vi "AlliGator Export ROI(s) NLSF Parameters as ASCII File.vi"(7 "AlliGator Ctrl Refnums":T2, 8 "error in (no error)":errorcluster, 10 "All ROIs":bool, 11 "AlliGator IV DVR in":refnum<data-value>) -> (0 "error out":errorcluster, 1 "Message":string, 3 "AlliGator IV DVR out":refnum<data-value>)   [LabVIEW 2021, in "AlliGator Decay Fit Parameter Map.lvlib"]
doc: "Exports Decay Fit Parameter Map data to an ASCII file."
uses:
  AlliGator Decay Fit Parameter Map.lvlib
  Strings/Strings.lvlib
  <userlib>/_OpenG.lib/array/array.llb/openg_array.lvlib
  AlliGator Variables List.ctl
  AlliGator Globals, Variables & Constants.lvlib
  Image/Named ROI Description.ctl
  Image/Image.lvlib
  <vilib>/Utility/file.llb/Write Delimited Spreadsheet (DBL).vi
  Fits/IRF(X)PSED/Decay Fit Parameters & Derived Quantities List.ctl
  Fits/Fits.lvlib
  <userlib>/_OpenG.lib/array/array.llb/Filter 1D Array with Scalar (String)__ogtk.vi
  <vilib>/vision/Image Controls.llb/IMAQ Image.ctl
  Phasor/Phasor Reference Series.ctl
  Phasor/Phasor.lvlib
  Phasor/Calibration Phasor (m, phi).ctl
  Phasor/Phasor (g, s).ctl
  AlliGator Baseline Subtraction Method.ctl
  AlliGator Decay Preprocessing.lvlib
  AlliGator Decay Background Subtraction Info.ctl
  AlliGator Decay Extrapolation Parameters.ctl
  AlliGator Decay Metadata v3.ctl
  AlliGator Phasor Graph.lvlib
  AlliGator Raw Phasor Plot Data v4.ctl
  AlliGator Data Series Type.ctl
  AlliGator Files.lvlib
  AlliGator Internal Variables v2.ctl
  AlliGator Internal Variables.lvlib
  AlliGator FLI Dataset Type.ctl
  Phasor/Phasor Harmonic Data.ctl
  AlliGator Phasor Multi-Harmonic Data.ctl
  AlliGator Phasor Plot.lvlib
  AlliGator Displayed Image.ctl
  AlliGator Source Image.lvlib
  Fits/IRF(X)PSED/Decay Fit Parameters In List.ctl
  AlliGator Decay Fit Parameter Constraints 2.ctl
  AlliGator Decay Fit.lvlib
  Fits/Decay Convolution/Decay Model.ctl
  Fits/Residual Type.ctl
  Fits/Fit Calculation Method.ctl
  Fits/Non-linear Fitting Algorithm.ctl
  AlliGator Decay Fit Options & Parameters v2.ctl
  Fits/IRF(X)PSED/Fit Weights Type.ctl
  AlliGator Gate Image Set.ctl
  AlliGator Gate Arithmetic.ctl
  AlliGator Settings.lvlib
  AlliGator Dataset Channel.ctl
  AlliGator Dual-Channel Datasets.lvlib
  AlliGator Registered Events Ctrl Refnums.ctl
  AlliGator GUI.lvlib
  AlliGator Dataset Ctrl Refnums.ctl
  Phasor/Phasor Calibration Type.ctl
  AlliGator Phasor Graph Ctrl Refnums.ctl
  AlliGator Phasor Plot Ctrl Refnums.ctl
  AlliGator State Indicator.ctl
  AlliGator Other Ctrl Refnums.ctl
  Histograms/Histogram Bin Position.ctl
  Histograms/Histogram Window.lvlib
  Histograms/Histogram Bin Option.ctl
  Histograms/Linear Histogram Options.ctl
  AlliGator Image Histogram Control Refnums.ctl
  AlliGator Decay Fit Map Control Refnums.ctl
  AlliGator Ctrl Refnums.ctl
  Graphs/XY Graph/XY Graph Plot Shift Method.ctl
  Graphs/XY Graph/XY Graph Add-Ons.lvlib
  Graphs/XY Graph/XY Graph Plot Shift Parameters.ctl
  AlliGator Decay Preprocessing Parameters.ctl
  Phasor/Phasor Standard Deviation Options.ctl
  Phasor/Phasor Calibration Map v2.ctl
  Fits/Non-linear Fitting Method v2.ctl
  Fits/IRF(X)PSED/Decay Fit Options v2.ctl
  Fits/IRF(X)PSED/MLE Baseline Offset Type.ctl
  AlliGator Parameter Maps Data.ctl
  AlliGator Main Window Tabs.ctl
panel:
  in  "Fit Parameter (for diagram use)":T1
  # "see the AlliGator License on the block diagram (Ctrl+E or Window:Show Block Diagram)"
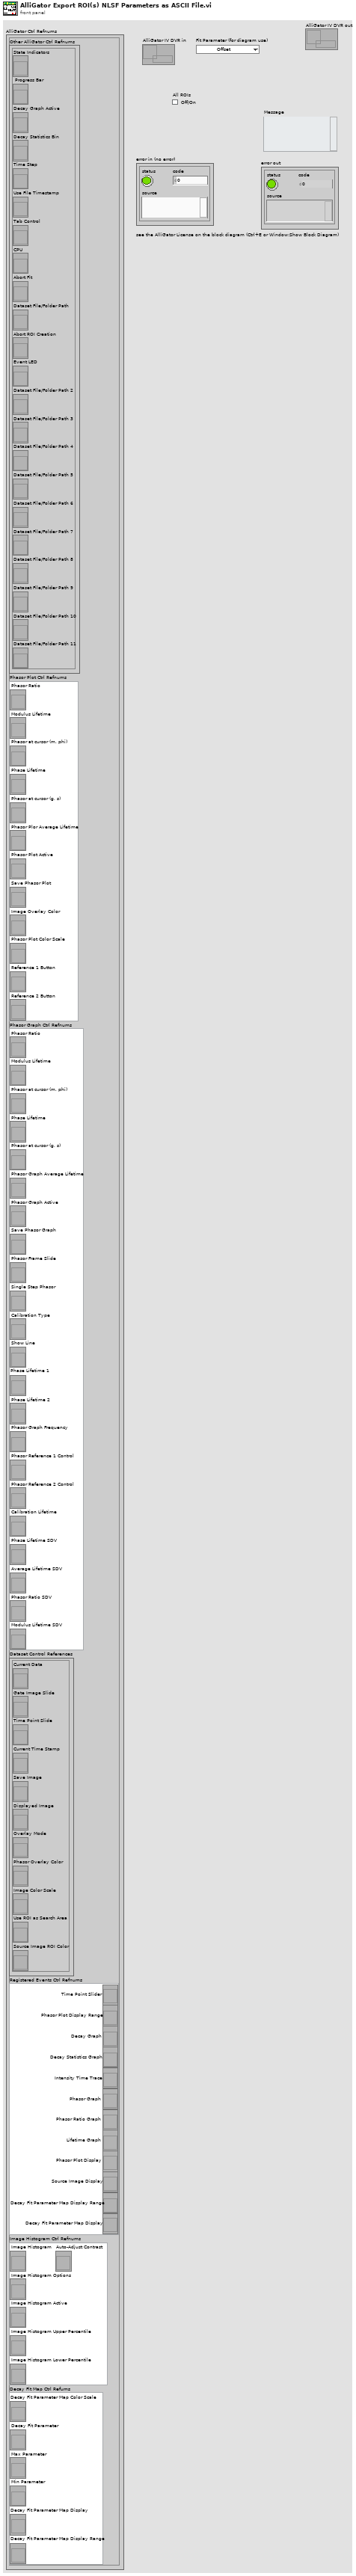
[diagram p1: front panel]
types:
  T1 = typedef "Fits.lvlib/Decay Fit Parameters & Derived Quantities List.ctl" = enum16{"Offset", "Baseline", "A_1", "tau_1", "A_2", "tau_2", "<tau>_a", "f1_a", "f2_a", "<tau>_i", "f1_i", "f2_i", "-", "R^2", "Chi^2"}
  T2 = typedef "AlliGator GUI.lvlib/AlliGator Ctrl Refnums.ctl" = cluster{"Other AlliGator Ctrl Refnums":T3, "Phasor Plot Ctrl Refnums":T4, "Phasor Graph Ctrl Refnums":T5, "Dataset Control References":T6, "Registered Events Ctrl Refnums":T7, "Image Histogram Ctrl Refnums":T8, "Decay Fit Map Ctrl Refums":T9}
  T3 = typedef "AlliGator GUI.lvlib/AlliGator Other Ctrl Refnums.ctl" = cluster{"State Indicators":refnum<vi>, " Progress Bar":refnum<vi>, "Decay Graph Active":refnum<vi>, "Decay Statistics Bin":refnum<vi>, "Time Step":refnum<vi>, "Use File Timestamp":refnum<vi>, "Tab Control":refnum<vi>, "CPU":refnum<vi>, "Abort Fit":refnum<vi>, "Dataset File/Folder Path":refnum<vi>, "Abort ROI Creation":refnum<vi>, "Event LED":refnum<vi>, "Dataset File/Folder Path 2":refnum<vi>, "Dataset File/Folder Path 3":refnum<vi>, "Dataset File/Folder Path 4":refnum<vi>, "Dataset File/Folder Path 5":refnum<vi>, "Dataset File/Folder Path 6":refnum<vi>, "Dataset File/Folder Path 7":refnum<vi>, "Dataset File/Folder Path 8":refnum<vi>, "Dataset File/Folder Path 9":refnum<vi>, "Dataset File/Folder Path 10":refnum<vi>, "Dataset File/Folder Path 11":refnum<vi>}
  T4 = typedef "AlliGator GUI.lvlib/AlliGator Phasor Plot Ctrl Refnums.ctl" = cluster{"Phasor Ratio":refnum<vi>, "Modulus Lifetime":refnum<vi>, "Phasor at cursor (m, phi)":refnum<vi>, "Phase Lifetime":refnum<vi>, "Phasor at cursor (g, s)":refnum<vi>, "Phasor Plor Average Lifetime":refnum<vi>, "Phasor Plot Active":refnum<vi>, "Save Phasor Plot":refnum<vi>, "Image Overlay Color":refnum<vi>, "Phasor Plot Color Scale":refnum<vi>, "Reference 1 Button":refnum<vi>, "Reference 2 Button":refnum<vi>}
  T5 = typedef "AlliGator GUI.lvlib/AlliGator Phasor Graph Ctrl Refnums.ctl" = cluster{"Phasor Ratio":refnum<vi>, "Modulus Lifetime":refnum<vi>, "Phasor at cursor (m, phi)":refnum<vi>, "Phase Lifetime":refnum<vi>, "Phasor at cursor (g, s)":refnum<vi>, "Phasor Graph Average Lifetime":refnum<vi>, "Phasor Graph Active":refnum<vi>, "Save Phasor Graph":refnum<vi>, "Phasor Frame Slide":refnum<vi>, "Single Step Phasor":refnum<vi>, "Calibration Type":refnum<vi>, "Show Line":refnum<vi>, "Phase Lifetime 1":refnum<vi>, "Phase Lifetime 2":refnum<vi>, "Phasor Graph Frequency":refnum<vi>, "Phasor Reference 1 Control":refnum<vi>, "Phasor Reference 2 Control":refnum<vi>, "Calibration Lifetime":refnum<vi>, "Phase Lifetime SDV":refnum<vi>, "Average Lifetime SDV":refnum<vi>, "Phasor Ratio SDV":refnum<vi>, "Modulus Lifetime SDV":refnum<vi>}
  T6 = typedef "AlliGator GUI.lvlib/AlliGator Dataset Ctrl Refnums.ctl" = cluster{"Current Data":refnum<vi>, "Gate Image Slide":refnum<vi>, "Time Point Slide":refnum<vi>, "Current Time Stamp":refnum<vi>, "Save Image":refnum<vi>, "Displayed Image":refnum<vi>, "Overlay Mode":refnum<vi>, "Phasor Overlay Color":refnum<vi>, "Image Color Scale":refnum<vi>, "Use ROI as Search Area":refnum<vi>, "Source Image ROI Color":refnum<vi>}
  T7 = typedef "AlliGator GUI.lvlib/AlliGator Registered Events Ctrl Refnums.ctl" = cluster{"Time Point Slider":refnum<vi>, "Phasor Plot Display Range":refnum<vi>, "Decay Graph":refnum<vi>, "Decay Statistics Graph":refnum<vi>, "Intensity Time Trace":refnum<vi>, "Phasor Graph":refnum<vi>, "Phasor Ratio Graph":refnum<vi>, "Lifetime Graph":refnum<vi>, "Phasor Plot Display":refnum<vi>, "Source Image Display":refnum<vi>, "Decay Fit Parameter Map Display Range":refnum<vi>, "Decay Fit Parameter Map Display":refnum<vi>}
  T8 = typedef "AlliGator GUI.lvlib/AlliGator Image Histogram Control Refnums.ctl" = cluster{"Image Histogram":refnum<vi>, "Image Histogram Options":refnum<vi>, "Image Histogram Active":refnum<vi>, "Image Histogram Upper Percentile":refnum<vi>, "Image Histogram Lower Percentile":refnum<vi>, "Auto-Adjust Contrast":refnum<vi>}
  T9 = typedef "AlliGator Decay Fit Parameter Map.lvlib/AlliGator Decay Fit Map Control Refnums.ctl" = cluster{"Decay Fit Parameter Map Color Scale":refnum<vi>, "Decay Fit Parameter":refnum<vi>, "Max Parameter":refnum<vi>, "Min Parameter":refnum<vi>, "Decay Fit Parameter Map Display":refnum<vi>, "Decay Fit Parameter Map Display Range":refnum<vi>}
  T10 = typedef "Image.lvlib/Named ROI Description.ctl" = cluster{"ROI Descriptor":T11, "ROI Name":string, "Overlay Color":u32}
  T11 = typedef "ROI Descriptor" = cluster{"Global Rectangle":i32[], "Contours":cluster{"ID":enum32{"External", "Internal"}, "Type":u32, "Coordinates":i32[]}[]}
  T12 = typedef "AlliGator Globals, Variables & Constants.lvlib/AlliGator Variables List.ctl" = enum16{"---- GUI ----", "GUI:Initialization Status", "GUI:State Indicators Refnum", "GUI:Original AlliGator Menu Items", "GUI:Current Action Loop State", "GUI:Script in progress", "GUI:Playback", "GUI:Loop Playback", "GUI:Search ROI Used", "GUI:Search ROI", "Decay Graph Max Legend Size", "Intensity Graph Max Legend Size", "Decay Statistics Graph Max Legend Size", "Phasor Graph Max Legend Size", "Phasor Ratio Graph Max Legend Size", "Lifetime Graph Max Legend Size", "---- Files ----", "Files:Export Dataset Frames as Individual Files", "Files:Show Batch Export Help Balloons", "Files:Frames in Dataset", "Files:ptu File Frame Start Indices", "Files:Current Frame in Dataset", "Files:Current Frame Timestamp", "Files:Dataset Loaded", "Files:Dataset Metadata", "Files:Dataset Channel", "Files:Dataset Data Description", "Files:Background Dataset Metadata", "Files:Background Dataset Channel", "Files:Background Dataset Data Description", "Files:Background File Subtraction", "Files:Background File Path", "Files:Background File Pile-up Correction", "Files:Background File Pixel Well Capacity", "Files:Background File Scaling Factor", "Files:Current Dataset Load Settings", "Files:Dataset Path", "Files:ICCD-specific Information", "Files:Macrotime Gate Separation", "------ Python Plugins ------", "Python Plugins:Information", "Python Plugins:Python Session", "Python Plugins:Valid Python Session?", "---- Source Image ----", "Source Image:ROIs", "Source Image:Current ROI", "Source Image:ROI Event Refnum", "X_Source Image Display Range", "X_Source Image Palette Information", "X_Type of Displayed Image", "X_Time Gate Slider", "Source Image:Palette List", "Source Image:Scale", "Source Image:ROI Overlay Color", "Source Image:Overlay to Erase", "Source Image:Is Displayed Image Accumulated", "Source Image:White Light Image Modified", "Source Image:Mask Image Modified", "---- Image Profile Window ----", "Image Profile:Overlay ROI in Source Image", "Image Profile:Window Event Refnum", "Image Profile:IntensityType", "Image Profile:Intensity Average Type", "Image Profile:Intensity-weighted SDV", "Image Profile:Box Profile Type", "Image Profile:Window Open", "Image Profile:Plotted Fit Parameter", "------ Phasor Graph -------", "Phasor Graph:Show Line", "---- Phasor Plot ---", "Phasor Plot:Parameters Changed", "Phasor Plot:FLI Dataset Modified since last Calculation", "Phasor Harmonics Data", "Selected Phasor Harmonics", "Phasor Harmonic Manager Event Refnum", "Phasor Plot:ROIs", "Phasor Plot:Current ROI", "Phasor Plot:ROI Event Refnum", "Phasor Plot:Image Reference Points", "Phasor Plot:Computed", "Phasor Plot:Palette Information", "Phasor Plot:Palette List", "Phasor Plot:Phasor Ratio Palette Information", "Phasor Plot:Phasor Ratio Palette List", "Phasor Plot:Image Scale", "Phasor Plot:Image Overlay to Erase", "Phasor Plot:Image Elements to Update", "Phasor Plot:Current Calculation Parameters", "Phasor Plot:Current Calibration Options", "Phasor Plot:Reset Cumulated Phasor Plot", "Phasor Plot:Reference 1", "Phasor Plot:Lifetime Reference 1", "Phasor Plot:Reference 1 Frequency", "Phasor Plot:Reference 2", "Phasor Plot:Lifetime Reference 2", "Phasor Plot:Reference 2 Frequency", "---- Decay Analysis ----", "Number of Selected Decays to Fit", "LS Fit Results", "LAR Fit Results", "BS Fit Results", "Last Decay Max - Min", "Best Fit Parameters", "Best Fit Parameter Names", "Actual Size X", "Actual Size Y", "Binning X", "Binning Y", "Actual # Gates", "Dataset Number", "Gates to...", "Gates Skipped", "Gates to keep", "Gate Step", "Gate Separation", "Reversed Gates", "Pile-up Correction", "Pixel Well Capacity", "Background Subtracted", "Background Subtraction Method", "Background Definition Range", "Background File (deprecated)", "Number of Dataset Accumulated", "Array of Accumulated Dataset Paths", "Do Averaged Datasets", "Destination File Path", "Process Plot Target", "Use 1/D as Phasor Frequency", "---- Decay Fit Parameter Map -----", "Decay Fit Parameter Map:Palette Information", "Decay Fit Parameter Map:Palette List", "------- Local Decay Window ---------", "Local Decay Graph Window:Event Refnum", "Local Decay Graph Window:Use normalized IRF for convolution", "----- Miscellaneous ----", "Misc:Skippable Dialog Windows Status"}
  T13 = typedef "AlliGator Internal Variables.lvlib/AlliGator Internal Variables v2.ctl" = cluster{"Displayed Image":T14, "White Light Image":T14, "Mask Image":T14, "ROI Mask Image":T14, "Current Dataset Images 1":T15, "Background Dataset Images 1":T15, "Current Dataset Images 2":T15, "Background Dataset Images 2":T15, "Current Dataset Arithmetic Images":T15, "Accumulated Dataset Images 1":T15, "Accumulated Dataset Images 2":T15, "Accumulated Dataset Arithmetic Images":T15, "Phasor Plot Image":T14, "Decay Fit Parameter Map Image":T14, "Single Data Point Path":path, "White Light Image Path":path, "Mask Image Path":path, "Time-Series Folder":path, "[Time-Series Paths]":path[], "Current Dataset":i32, "Single Dataset Type":T16, "Current Folder":string, "AlliGator Data Series Type":T17, "# Datasets":i32, "Dual-Channel Dataset":bool, "Selected Channel Name":string, "Dataset Channel":T18, "Channel Arithmetic":T19, "Dual-Channel Background Dataset":bool, "Background Channel":T18, "Dual-Channel Accumulated Dataset":bool, "Start Time":dbl, "[Time-Series Timestamps]":dbl[], "[Intensity Corrections]":dbl[], "Time Series Script":bool, "Type of Displayed Image":T20, "Gate Image Slide":u16, "# Gates":i32, "ROIs":T10[], "ROI Decay":cluster{"t Array":dbl[], "I Array":dbl[]}, "Valid Decay":bool, "Decay  Metadata":T21, "Reference Decay Plot Name":string, "Reference Decay":cluster{"t Array":dbl[], "I Array":dbl[]}, "Decay Shift Plot":cluster{"Time Stamps":dbl[], "Decay Shifts":dbl[]}, "[Decays Max Values]":sgl[], "[Decays Min Values]":sgl[], "Calibration Phasor":T27, "Calibration Phasor Series":T28, "Phasor Calibration Map":T29, "Calibration Map MD5 Digest":string, "Last Raw Phasor":T30, "Last Calibrated Phasor":T30, "Last Calibrated Phasor SDV":T30, "Phasor Graph:Phasor Plot":cluster{"g Array":dbl[], "s Array":dbl[]}, "Phasor Graph:Phasor SDV Plot":cluster{"g Array":dbl[], "s Array":dbl[]}, "[Phasor Graph:Raw Phasor Plots]":T31[], "Phasor Plot locked to Ref 1":i32, "[Phasor Plot(s) locked to Ref 1]":i32[], "[Phasor Plot(s) locked to Ref 2]":i32[], "[Pixel Phasors]":T30[], "[[Sum Image]]":dbl[][], "[[CSG Phasors]]":csg[][], "[[Valid Pixel?]]":bool[][], "I/m/phi Dataset":cluster{"I/m/phi Dataset?":bool, "Base Frequency":dbl[unit], "Harmonic Orders":u8[]}, "Multi Phasor Plot Data":T33, "Decay Fit Options & Parameters":T35, "Fit Options: Decay Preprocessing Parameters":T46, "Fit Options: Reference Decay":cluster{"t Array":dbl[], "I Array":dbl[]}, "Is Full Image Parameters Map":bool, "Is Single-Pixels Parameters Map":bool, "NLSF Parameters Map X Resolution":i32, "NLSF Parameters Map Y Resolution":i32, "[Single Decay Fit Parameters]":dbl[], "Fit Model":T37, "[[Multiple Decays Fit Parameters]]":dbl[][], "[[Multiple Decays Fit Parameter SDVs]]":dbl[][], "[[IRFs]]":dbl[][], "IRF Array Time Axis":dbl[], "Decay Array Time Axis":dbl[], "[Decay Fit Parameter Names]":T1[], "[[Phasor Ratios]]":dbl[][], "[[Average Lifetimes]]":dbl[][], "Amplitude Weighted Average Lifetime":bool, "[Decay Sum]":dbl[], "Parameter Maps":T47[], "[[User-defined Quantities]]":dbl[][], "User-defined Quantity":string}
  T14 = typedef "IMAQ Image.ctl" = refnum<image>
  T15 = typedef "AlliGator Internal Variables.lvlib/AlliGator Gate Image Set.ctl" = cluster{"SGL Image Max":T14, "SGL Image Sum":T14, "SGL Gate Images":T14[], "SGL Image Min":T14}
  T16 = typedef "AlliGator Files.lvlib/AlliGator FLI Dataset Type.ctl" = enum16{"HDF5 FLI Dataset", "Gate Image Folder", ".sdt FLI Dataset (Becker & Hickl)", ".ptu FLI Dataset (PicoQuant)", "SS1 FLI Dataset", "SS2 FLI Dataset", "I/m/phi Dataset", ".bin FLI Dataset (PicoQuant Binned)", ".bin FLI Dataset (Piccolo Binned)"}
  T17 = typedef "AlliGator Files.lvlib/AlliGator Data Series Type.ctl" = enum16{"Not a Supported Series", "Gate Images Folder Series", "SwissSPAD 2 Dataset Series", "B&H FLI Dataset Series", "PicoQuant PTU FLI Dataset Series", "PicoQuant BIN FLI Dataset Series", "Piccolo hist BIN FLI Dataset Series", "HDF5 FLI Dataset Series"}
  T18 = typedef "AlliGator Dual-Channel Datasets.lvlib/AlliGator Dataset Channel.ctl" = enum16{"G2", "INT"}
  T19 = typedef "AlliGator Settings.lvlib/AlliGator Gate Arithmetic.ctl" = enum16{"None", "INT-G2", "G2/INT*<INT>", "(1 - G2/INT)*<INT>"}
  T20 = typedef "AlliGator Source Image.lvlib/AlliGator Displayed Image.ctl" = enum16{"Single Gate", "Sum of All Gates", "Max of All Gates", "Min of All Gates", "-", "White Ligth Image", "Mask Image"}
  T21 = typedef "AlliGator Phasor Graph.lvlib/AlliGator Decay Metadata v3.ctl" = cluster{"ROI Descriptor":T11, "ROI Center":cluster{"X":i32, "Y":i32}, "Decay Background Subtraction Info":T22, "Decay Reverted":bool, "Decay Smoothened":bool, "Decay Straightened":bool, "Fitted Tau (Decay Straightening)":dbl, "Decay Shift Parameters":T24, "Decay Shifted":bool, "Decay Extrapolated":bool, "Decay Extrapolation Parameters":T26, "Decay Normalized":bool, "Fold Decay":bool, "# Folds":u32}
  T22 = typedef "AlliGator Decay Analysis.lvlib/AlliGator Decay Preprocessing.lvlib/AlliGator Decay Background Subtraction Info.ctl" = cluster{"Laser Period":dbl[unit], "Gate Duration":dbl[unit], "Baseline Subtraction Method":T23, "Background Definition Range":cluster{"Min Gate":dbl[unit], "Max Gate":dbl[unit]}, "Total Intensity w/o Bkgd Subtraction":dbl, "Bkgd-subtracted Intensity (exp)":dbl, "# Data Points":i32, "Background/Gate":dbl, "Fitted Lifetime":dbl[unit], "Bkgd-subtracted Intensity (theo)":dbl}
  T23 = typedef "AlliGator Decay Analysis.lvlib/AlliGator Decay Preprocessing.lvlib/AlliGator Baseline Subtraction Method.ctl" = enum16{"Mean", "Min", "Square Gated Single-Exponential", "File", "Constant"}
  T24 = typedef "XY Graph Add-Ons.lvlib/XY Graph Plot Shift Parameters.ctl" = cluster{"Type":T25, "Shift":dbl[unit], "Threshold":dbl, "Rotate":bool}
  T25 = typedef "XY Graph Add-Ons.lvlib/XY Graph Plot Shift Method.ctl" = enum16{"Default", "CFD", "Threshold", "Cross-Correlation"}
  T26 = typedef "AlliGator Decay Analysis.lvlib/AlliGator Decay Preprocessing.lvlib/AlliGator Decay Extrapolation Parameters.ctl" = cluster{"Additional Points":u32, "Head Fraction":dbl, "Fitted Tau":dbl, "Use Periodicity":bool, "Use Cursors":bool, "Tail Fraction":dbl}
  T27 = typedef "Phasor.lvlib/Calibration Phasor (m, phi).ctl" = cluster{"m":dbl, "phi":dbl, "Phasor Frequency":dbl[unit], "Reference Lifetime":dbl[unit]}
  T28 = typedef "Phasor.lvlib/Phasor Reference Series.ctl" = cluster{"m Array":dbl[], "phi Array":dbl[], "Phasor Frequency":dbl[unit], "Calibration Lifetime":dbl[unit]}
  T29 = typedef "Phasor.lvlib/Phasor Calibration Map v2.ctl" = cluster{"Phasor Frequency":dbl[unit], "Calibration Lifetime":dbl[unit], "ROI Centers":cluster{"X":i32, "Y":i32}[], "ROI Descriptors":T11[], "Map Resolution X":i32, "Map Resolution Y":i32, "z Array":cdb[]}
  T30 = typedef "Phasor.lvlib/Phasor (g, s).ctl" = cluster{"g":dbl, "s":dbl}
  T31 = typedef "AlliGator Phasor Graph.lvlib/AlliGator Raw Phasor Plot Data v4.ctl" = cluster{"Phasor Plot Name":string, "Raw Phasor Plot":T30[], "Phasor Frequency":dbl[unit], "[Decay Metadata]":T21[], "Raw Phasor Plot SDV":T30[], "Phasor SDV Options":T32, "[Calibration Phasor]":T27[]}
  T32 = typedef "Phasor.lvlib/Phasor Standard Deviation Options.ctl" = cluster{"Compute Estimated SDV":bool, "# Replicas":u32, "Use Estimated Average Phasor":bool}
  T33 = typedef "AlliGator Phasor Plot.lvlib/AlliGator Phasor Multi-Harmonic Data.ctl" = cluster{"Base Frequency":dbl[unit], "# Harmonics":u8, "Harmonic Orders":u8[], "Phasor Plot Settings Checksum":u64, "Phasor Harmonic Data Array":T34[]}
  T34 = typedef "Phasor.lvlib/Phasor Harmonic Data.ctl" = cluster{"Phasor Harmonic Name":string, "Phasor Plot Settings Checksum":u64, "Phasor Frequency":dbl[unit], "Base Frequency":dbl[unit], "Harmonic Order":u8, "Phasor Plot Parameters":string, "Phasor Array [[CSG]]":csg[][], "Dataset File Path":path}
  T35 = typedef "AlliGator Decay Fit Parameter Map.lvlib/AlliGator Decay Fit Options & Parameters v2.ctl" = cluster{"SYNC Period":dbl[unit], "Fit Options":T36, "Fit Parameter Constraints":T43[], "MLE Baseline Offset":dbl, "MLE Baseline Offset Type":T45}
  T36 = typedef "Fits.lvlib/Decay Fit Options v2.ctl" = cluster{"Show Fit Residuals":bool, "Fit Model":T37, "Residual Type":T38, "Max Decay Percentile":dbl, "Min Decay Percentile":dbl, "Show Full Decay":bool, "Weights":T39, "Fitting Method":T40, "Compute Parameter Uncertainties":bool, "Periodic Boundaries":bool, "Model Calculation":T41, "Period":dbl[unit], "Termination Criteria":cluster{"Max Iterations":i32, "Max Function Calls":i32, "Max Time":dbl[unit], "Function Tolerance":dbl, "Parameter Tolerance":dbl, "Gradient Tolerance":dbl, "Min Lambda":dbl, "Max Lambda":dbl, "Initial Tick Count":u32}, "Offset Resolution":dbl[unit], "Use Local IRF":bool, "Fitting Algorithm":T42}
  T37 = typedef "Fits.lvlib/Decay Model.ctl" = enum16{"1-Exponential", "2-Exponentials"}
  T38 = typedef "Fits.lvlib/Residual Type.ctl" = enum16{"Standard", "Normalized", "Reduced"}
  T39 = typedef "Fits.lvlib/Fit Weights Type.ctl" = enum16{"Unweighted", "1/Variance", "Best of All"}
  T40 = typedef "Fits.lvlib/Non-linear Fitting Method v2.ctl" = enum16{"Least Square", "Least Absolute Residual", "Bisquare", "MLE", "-", "Best of All"}
  T41 = typedef "Fits.lvlib/Fit Calculation Method.ctl" = enum16{"Simulation", "Convolution", "Integration"}
  T42 = typedef "Fits.lvlib/Non-linear Fitting Algorithm.ctl" = enum16{"Levenberg-Marquardt", "Trust-Region Dogleg"}
  T43 = typedef "AlliGator Decay Analysis.lvlib/AlliGator Decay Fit.lvlib/AlliGator Decay Fit Parameter Constraints 2.ctl" = cluster{"Fit Parameter":T44, "Min Value":dbl, "Max Value":dbl, "Global":bool, "Used":bool}
  T44 = typedef "Fits.lvlib/Decay Fit Parameters In List.ctl" = enum16{"Offset", "Baseline", "A_1", "tau_1", "A_2", "tau_2"}
  T45 = typedef "Fits.lvlib/MLE Baseline Offset Type.ctl" = enum32{"Absolute", "Percentage"}
  T46 = typedef "AlliGator Decay Analysis.lvlib/AlliGator Decay Preprocessing.lvlib/AlliGator Decay Preprocessing Parameters.ctl" = cluster{"Background Subtraction":bool, "Straighten Decay":bool, "Reverse Gates":bool, "1-Normalized Decay":bool, "Smoothen Decay":bool, "Smoothing Parameter":dbl, "Shift Decay":bool, "Decay Shift Parameters":T24, "Extrapolate Decay":bool, "Additional Points":u32, "Head Fraction":dbl, "Pixel-Normalize Decay":bool, "Use Periodicity":bool, "Use Cursors":bool, "Tail Fraction":dbl, "Use Decay Pre-Processing":bool, "Fold Decay":bool, "# Folds":u32, "[0-1]-Normalized Decay":bool}
  T47 = typedef "AlliGator Parameter Maps Data.ctl" = cluster{"Map Set Name":string, "[Parameter Names]":string[], "[[Parameters]]":dbl[][], "[[Parameter SDVs]]":dbl[][], "Decay Array Time Axis":dbl[], "[[IRFs]]":dbl[][], "IRF Array Time Axis":dbl[]}
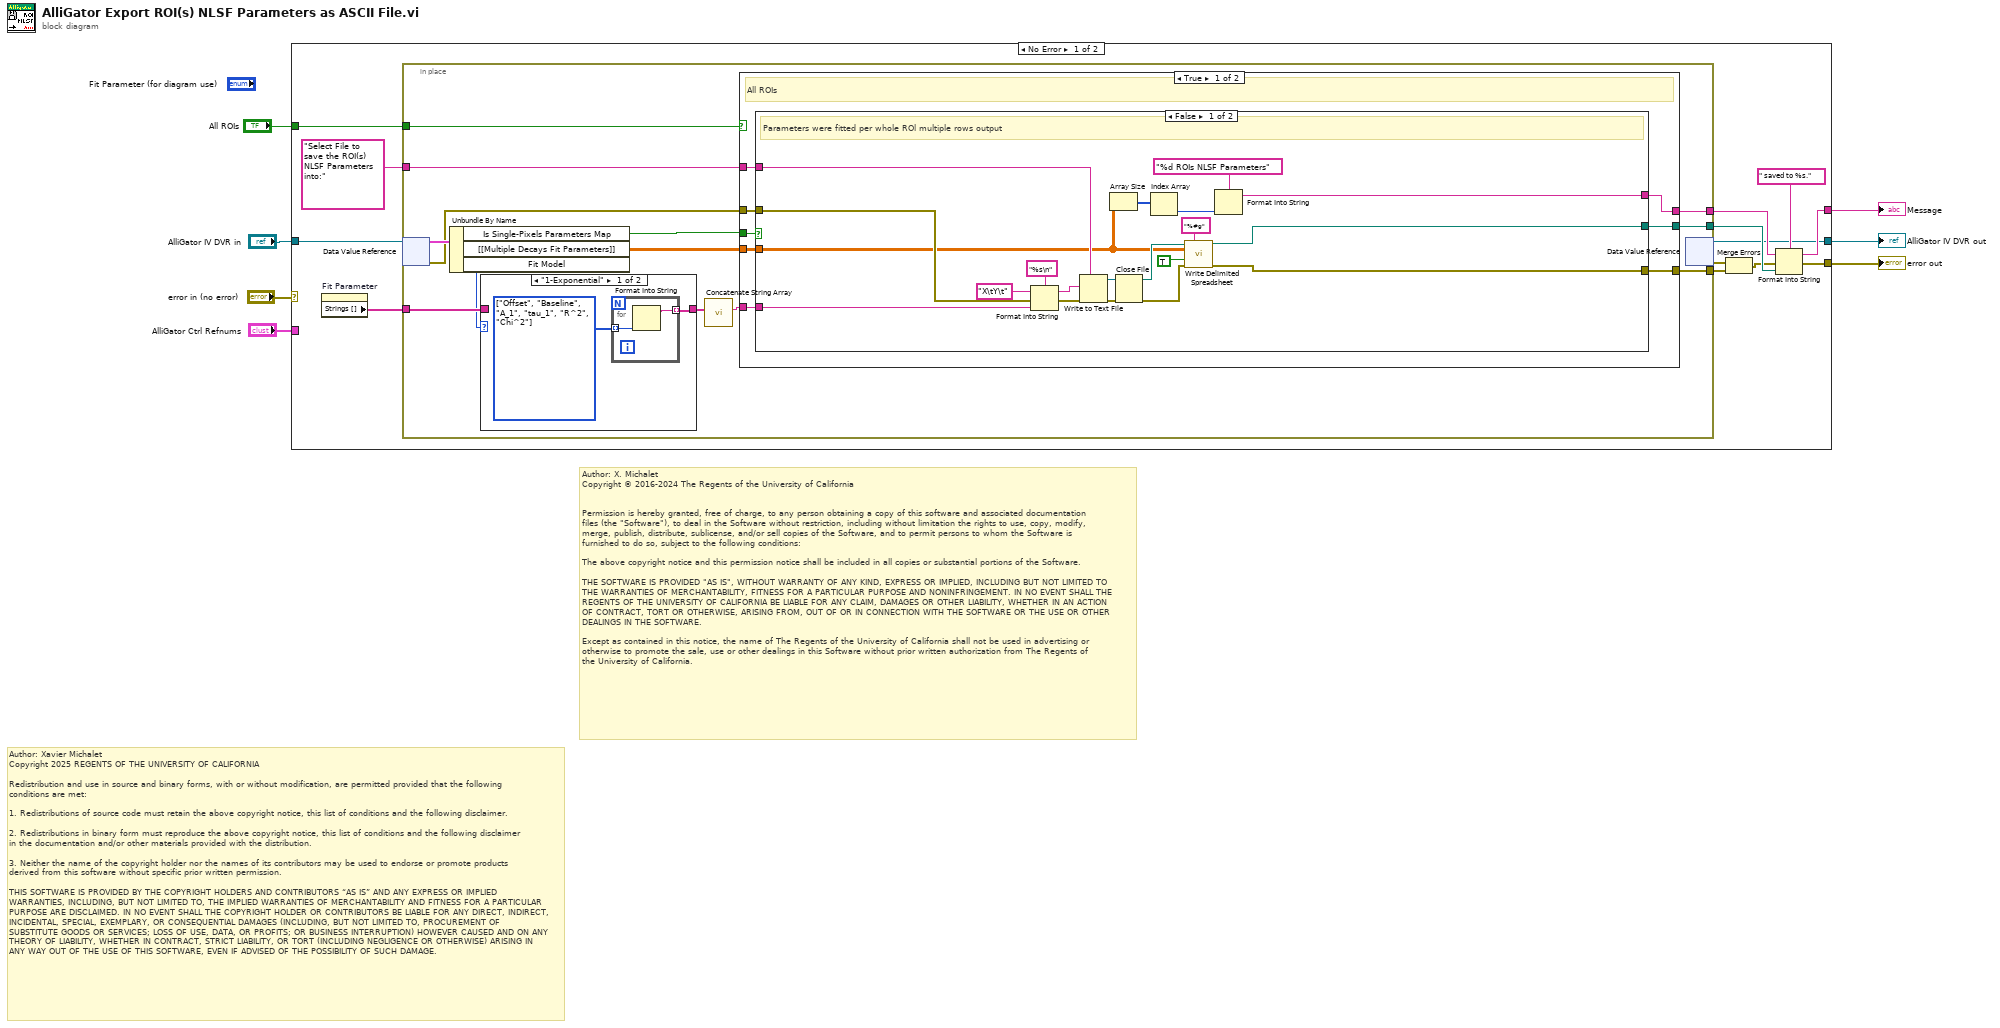
[diagram p0: block diagram]
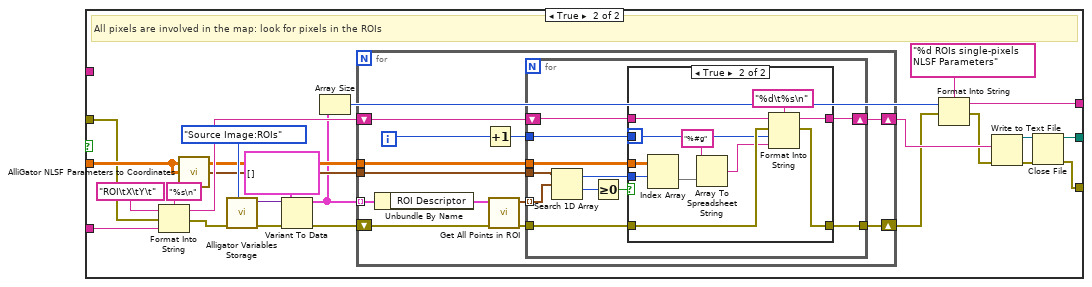
[diagram p2: hidden frame]
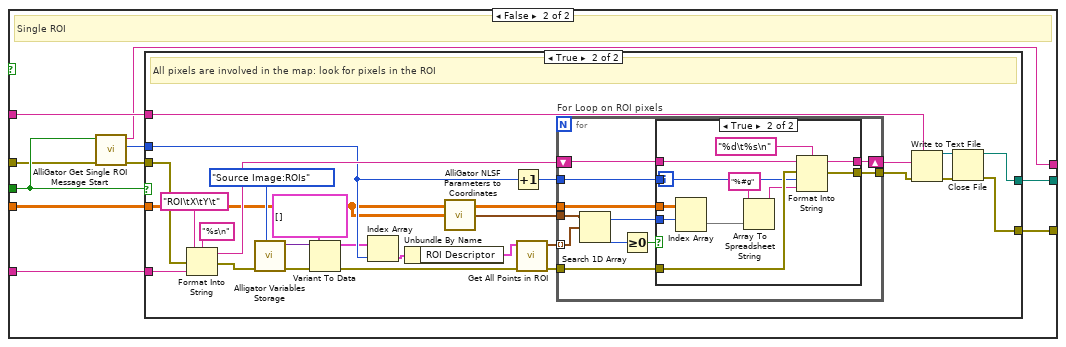
[diagram p4: hidden frame]
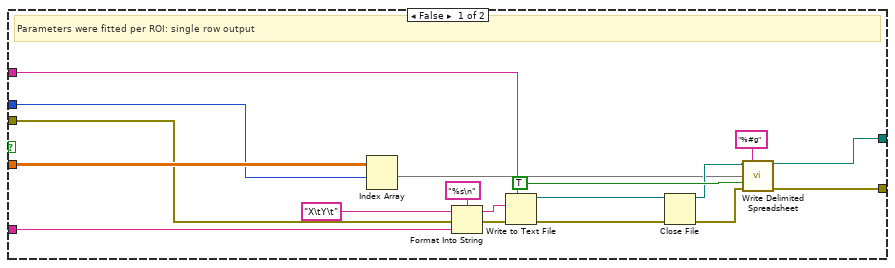
[diagram p5: hidden frame]
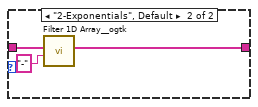
[diagram p7: hidden frame]
diagram:
  # "Author: Xavier Michalet\nCopyright 2025 REGENTS OF THE UNIVERSITY OF CALIFORNIA\n\nRedistribution and use in source and binary forms, with or without modification, are permitted provided that the following conditions are met:\n\n1. Redistributions of source code must retain the above copyright notice, this list of conditions and the following disclaimer.\n\n2. Redistributions in binary form must reproduce the above copyright notice, this list of conditions and the following disclaimer in the documentation and/or other materials provided with the distribution.\n\n3. Neither the name of the copyright holder nor the names of its contributors may be used to endorse or promote products derived from this software without specific prior written permission.\n\nTHIS SOFTWARE IS PROVIDED BY THE COPYRIGHT HOLDERS AND CONTRIBUTORS “AS IS” AND ANY EXPRESS OR IMPLIED WARRANTIES, INCLUDING, BUT NOT LIMITED TO, THE IMPLIED WARRANTIES OF MERCHANTABILITY AND FITNESS FOR A PARTICULAR PURPOSE ARE DISCLAIMED. IN NO EVENT SHALL THE COPYRIGHT HOLDER OR CONTRIBUTORS BE LIABLE FOR ANY DIRECT, INDIRECT, INCIDENTAL, SPECIAL, EXEMPLARY, OR CONSEQUENTIAL DAMAGES (INCLUDING, BUT NOT LIMITED TO, PROCUREMENT OF SUBSTITUTE GOODS OR SERVICES; LOSS OF USE, DATA, OR PROFITS; OR BUSINESS INTERRUPTION) HOWEVER CAUSED AND ON ANY THEORY OF LIABILITY, WHETHER IN CONTRACT, STRICT LIABILITY, OR TORT (INCLUDING NEGLIGENCE OR OTHERWISE) ARISING IN ANY WAY OUT OF THE USE OF THIS SOFTWARE, EVEN IF ADVISED OF THE POSSIBILITY OF SUCH DAMAGE."
  # "Author: X. Michalet\nCopyright © 2016-2024 The Regents of the University of California\n \n\nPermission is hereby granted, free of charge, to any person obtaining a copy of this software and associated documentation files (the \"Software\"), to deal in the Software without restriction, including without limitation the rights to use, copy, modify, merge, publish, distribute, sublicense, and/or sell copies of the Software, and to permit persons to whom the Software is furnished to do so, subject to the following conditions:\n\nThe above copyright notice and this permission notice shall be included in all copies or substantial portions of the Software.\n\nTHE SOFTWARE IS PROVIDED \"AS IS\", WITHOUT WARRANTY OF ANY KIND, EXPRESS OR IMPLIED, INCLUDING BUT NOT LIMITED TO THE WARRANTIES OF MERCHANTABILITY, FITNESS FOR A PARTICULAR PURPOSE AND NONINFRINGEMENT. IN NO EVENT SHALL THE REGENTS OF THE UNIVERSITY OF CALIFORNIA BE LIABLE FOR ANY CLAIM, DAMAGES OR OTHER LIABILITY, WHETHER IN AN ACTION OF CONTRACT, TORT OR OTHERWISE, ARISING FROM, OUT OF OR IN CONNECTION WITH THE SOFTWARE OR THE USE OR OTHER DEALINGS IN THE SOFTWARE.\n\nExcept as contained in this notice, the name of The Regents of the University of California shall not be used in advertising or otherwise to promote the sale, use or other dealings in this Software without prior written authorization from The Regents of the University of California."
  n1 = case shown="No Error" "error in (no error)" {
    selector: "error in (no error)" -> [_ w207]
    tunnel: "AlliGator Ctrl Refnums" -> [_ _]
    tunnel: [w12 w206] -> w6
    tunnel: "AlliGator IV DVR in" -> [w13 w206]
    tunnel: [w18 w207] -> w4
    tunnel: "All ROIs" -> [w20 _]
    tunnel: [w17 _] -> w1
    frame No Error {
      n2 = property on="Fit Parameter" class="Enum (strict)"() -> ("Strings []"=w8:string[])  [unwired: 2 in, 2 out]
      n3 = in-place {
        in-place-border: w20 -> [w33]
        in-place-border: "Select File to save the ROI(s) NLSF Parameters into:" ("prompt (Choose or enter file path)") -> [w32]
        in-place-border: [w31] -> w16
        in-place-border: [w30] -> w14
        in-place-border: [w25] -> w10
        in-place-border: w8 -> [w24]
        n4 = in-place-dvr #1(w13) -> (w29:T13, w26:errorcluster)
        n5 = Unbundle By Name(w29) -> ("Is Single-Pixels Parameters Map"=w28:bool, "[[Multiple Decays Fit Parameters]]"=w27:dbl[][], "Fit Model"=w23:T37)
        n6 = case shown="\"1-Exponential\"" w23 {
          tunnel: w24 -> [_ w204]
          tunnel: [w199 w203] -> w22
          frame "1-Exponential" {
            w200 = T1[] [enum."Offset", enum."Baseline", enum."A_1", enum."tau_1", enum."R^2", enum."Chi^2"] items=["Offset", "Baseline", "A_1", "tau_1", "A_2", "tau_2", "<tau>_a", "f1_a", "f2_a", "<tau>_i", "f1_i", "f2_i", "-", "R^2", "Chi^2"] ("t")
            n7 = for {
              tunnel: w200 -> [w202] mode=indexing
              tunnel: [w201] -> w199 mode=indexing
              n8 = Format Into String(w202) -> (resulting string=w201:string)  [unwired: 3 in, 1 out]
            }
          }
          frame "2-Exponentials", Default {
            n9 = call-poly <userlib>:"Filter 1D Array__ogtk.vi"("items to filter"="-", "array"=w204) -> ("filtered array"=w203:string[])  [unwired: 4 in, 1 out]
          }
        }
        n10 = call "Concatenate String Array.vi"("String Array"=w22) -> ("Formatted String"=w21:string)  [unwired: 10 in]
        n11 = case shown="True" w33 {
          tunnel: [w41 w130] -> w31
          tunnel: [w40 w129] -> w25
          tunnel: w32 -> [w39 w128]
          tunnel: w21 -> [w38 w127]
          tunnel: [w37 w126] -> w30
          tunnel: w28 -> [w36 w125]
          tunnel: w27 -> [w35 w124]
          tunnel: w26 -> [w34 w121]
          frame True {
            # "All ROIs"
            n12 = case shown="False" w36 {
              tunnel: w35 -> [w46 w72]
              tunnel: w34 -> [w54 w62]
              tunnel: [w59 w70] -> w41
              tunnel: [w58 w71] -> w40
              tunnel: w39 -> [w56 _]
              tunnel: w38 -> [w55 w63]
              tunnel: [w42 w66] -> w37
              frame False {
                # "Parameters were fitted per whole ROl multiple rows output"
                n13 = Format Into String(format string="%s\n", initial string="X\tY\t", error in=w54, w55) -> (resulting string=w52:string, error out=w53:errorcluster)
                n14 = Write to Text File(prompt (Choose or enter file path)=w56, text=w52, error in=w53) -> (refnum out=w48:refnum<file>, error out=w57:errorcluster)  [unwired: 1 in, 1 out]
                n15 = Array Size(array=w46) -> (size(s)=w45:i32[])
                n16 = Close File(refnum=w48, error in=w57) -> (path=w47:path, error out=w49:errorcluster)
                n17 = Index Array(array=w45) -> (element=w44:i32)  [unwired: 1 in]
                n18 = call-poly <vilib>:"Write Delimited Spreadsheet.vi"("file path (dialog if empty)"=w47, "format (%.3f)"="%#g", "2D data"=w46, "append to file? (new file:F)"=TRUE, "error in (no error)"=w49) -> ("new file path (Not A Path if cancelled)"=w59:path, "error out"=w58:errorcluster)  [unwired: 9 in]
                n19 = Format Into String(format string="%d ROIs NLSF Parameters", w44) -> (resulting string=w42:string)  [unwired: 2 in, 1 out]
              }
              frame True {
                # "All pixels are involved in the map: look for pixels in the ROIs"
                n20 = Format Into String(format string="%s\n", initial string="ROI\tX\tY\t", error in=w62, w63) -> (resulting string=w79:string, error out=w80:errorcluster)
                n21 = call "AlliGator NLSF Parameters to Coordinates.vi"("[[Multiple Decays Fit Parameters]]"=w72) -> ("Decay Locations"=w73:cluster{"X":i32, "Y":i32}[])
                n22 = call "Alligator Variables Storage.vi"("AlliGator Variable"=AlliGator_Variables_List."Source Image:ROIs" ("Alligator Variable"), "Error In"=w80) -> ("Error Out"=w83:errorcluster, "Data out"=w74:variant)  [unwired: 7 in, 1 out]
                n23 = Variant To Data(error in=w83, type=T10[] [] ("Stored ROIs in"), Variant=w74) -> (data=w69:T10[], error out=w75:errorcluster)
                n24 = Array Size(array=w69) -> (size(s)=w68:i32)
                n25 = for {
                  tunnel: w73 -> [w89]
                  shift-right: [w96] -> w78
                  shift-left: w79 -> [w97]
                  shift-right: [w95] -> w65
                  shift-left: w75 -> [w92]
                  tunnel: w69 -> [w88] mode=indexing
                  tunnel: w72 -> [w86]
                  i -> [w87]
                  n26 = Unbundle By Name(w88) -> ("ROI Descriptor"=w93:T11)
                  n27 = Increment(x=w87) -> (x+1=w94:i32)
                  n28 = call "Get All Points in ROI.vi"("Error In"=w92, "ROI Descriptor"=w93) -> ("Error Out"=w91:errorcluster, "Point Array"=w90:cluster{"X":i32, "Y":i32}[])  [unwired: 8 in]
                  n29 = for {
                    tunnel: w91 -> [w105]
                    shift-right: [w106] -> w96
                    shift-left: w97 -> [w107]
                    tunnel: [w104] -> w95
                    tunnel: w94 -> [w103]
                    tunnel: w90 -> [w102] mode=indexing
                    tunnel: w89 -> [w99]
                    tunnel: w86 -> [w98]
                    n30 = Search 1D Array(1D array=w99, element=w102) -> (index of element=w101:i32)  [unwired: 1 in]
                    n31 = Greater Or Equal To 0?(x=w101) -> (x >= 0?=w100:bool)
                    n32 = case shown="True" w100 {
                      tunnel: w107 -> [w109 w120]
                      tunnel: [w109 w119] -> w106
                      tunnel: w105 -> [w108 w117]
                      tunnel: [w108 w116] -> w104
                      tunnel: w103 -> [_ w115]
                      tunnel: w101 -> [_ w112]
                      tunnel: w98 -> [_ w111]
                      frame False {
                        # "No good fit at that pixel"
                      }
                      frame True {
                        n33 = Index Array(array=w111, index (row)=w112) -> (element=w110:dbl[])  [unwired: 1 in]
                        n34 = Array To Spreadsheet String(array=w110, 3:"%#g" ("format string")) -> (spreadsheet string=w113:string)  [unwired: 1 in]
                        n35 = Format Into String(format string="%d\t%s\n", initial string=w120, error in=w117, w115, w113) -> (resulting string=w119:string, error out=w116:errorcluster)
                      }
                    }
                  }
                }
                n36 = Format Into String(format string="%d ROIs single-pixels NLSF Parameters", error in=w65, w68) -> (resulting string=w66:string, error out=w64:errorcluster)  [unwired: 1 in]
                n37 = Write to Text File(text=w78, error in=w64) -> (refnum out=w76:refnum<file>, error out=w77:errorcluster)  [unwired: 2 in, 1 out]
                n38 = Close File(refnum=w76, error in=w77) -> (path=w70:path, error out=w71:errorcluster)
              }
            }
          }
          frame False {
            # "Single ROI"
            n39 = call "AlliGator Get Single ROI Message Start.vi"("error in (no error)"=w121, "Single-Pixel Fit?"=w125) -> ("error out"=w123:errorcluster, "ROI idx"=w122:i32, "Message header"=w126:string)  [unwired: 7 in]
            n40 = case shown="True" w125 {
              tunnel: w124 -> [w134 w150]
              tunnel: [w146 w161] -> w130
              tunnel: [w145 w162] -> w129
              tunnel: w128 -> [w143 w160]
              tunnel: w127 -> [w142 w175]
              tunnel: w123 -> [w132 w168]
              tunnel: w122 -> [w131 w159]
              frame False {
                # "Parameters were fitted per ROI: single row output"
                n41 = Index Array(array=w134, index (row)=w131) -> (element=w133:dbl[])  [unwired: 1 in]
                n42 = Format Into String(format string="%s\n", initial string="X\tY\t", error in=w132, w142) -> (resulting string=w140:string, error out=w141:errorcluster)
                n43 = Write to Text File(prompt (Choose or enter file path)=w143, text=w140, error in=w141) -> (refnum out=w136:refnum<file>, error out=w144:errorcluster)  [unwired: 1 in, 1 out]
                n44 = Close File(refnum=w136, error in=w144) -> (path=w135:path, error out=w137:errorcluster)
                n45 = call-poly <vilib>:"Write Delimited Spreadsheet.vi"("file path (dialog if empty)"=w135, "format (%.3f)"="%#g", "1D data"=w133, "append to file? (new file:F)"=TRUE, "error in (no error)"=w137) -> ("new file path (Not A Path if cancelled)"=w146:path, "error out"=w145:errorcluster)  [unwired: 9 in]
              }
              frame True {
                # "All pixels are involved in the map: look for pixels in the ROI"
                n46 = Format Into String(format string="%s\n", initial string="ROI\tX\tY\t", error in=w168, w175) -> (resulting string=w167:string, error out=w169:errorcluster)
                n47 = call "Alligator Variables Storage.vi"("AlliGator Variable"=AlliGator_Variables_List."Source Image:ROIs" ("Alligator Variable"), "Error In"=w169) -> ("Error Out"=w172:errorcluster, "Data out"=w152:variant)  [unwired: 7 in, 1 out]
                n48 = Variant To Data(error in=w172, type=T10[] [] ("Stored ROIs in"), Variant=w152) -> (data=w151:T10[], error out=w155:errorcluster)
                n49 = Index Array(array=w151, index=w159) -> (element=w157:T10)
                n50 = Unbundle By Name(w157) -> ("ROI Descriptor"=w156:T11)
                n51 = call "AlliGator NLSF Parameters to Coordinates.vi"("[[Multiple Decays Fit Parameters]]"=w150) -> ("Decay Locations"=w149:cluster{"X":i32, "Y":i32}[])
                n52 = Increment(x=w159) -> (x+1=w158:i32)
                n53 = call "Get All Points in ROI.vi"("Error In"=w155, "ROI Descriptor"=w156) -> ("Error Out"=w154:errorcluster, "Point Array"=w153:cluster{"X":i32, "Y":i32}[])  [unwired: 8 in]
                n54 = for "For Loop on ROI pixels" {
                  tunnel: w154 -> [w183]
                  shift-right: [w184] -> w166
                  shift-left: w167 -> [w185]
                  tunnel: [w182] -> w165
                  tunnel: w158 -> [w181]
                  tunnel: w150 -> [w180]
                  tunnel: w153 -> [w179] mode=indexing
                  tunnel: w149 -> [w176]
                  n55 = Search 1D Array(1D array=w176, element=w179) -> (index of element=w178:i32)  [unwired: 1 in]
                  n56 = Greater Or Equal To 0?(x=w178) -> (x >= 0?=w177:bool)
                  n57 = case shown="True" w177 {
                    tunnel: w185 -> [w187 w198]
                    tunnel: [w187 w197] -> w184
                    tunnel: w183 -> [w186 w195]
                    tunnel: [w186 w194] -> w182
                    tunnel: w181 -> [_ w193]
                    tunnel: w180 -> [_ w192]
                    tunnel: w178 -> [_ w188]
                    frame False {
                      # "No good fit at that pixel"
                    }
                    frame True {
                      n58 = Index Array(array=w192, index (row)=w188) -> (element=w189:dbl[])  [unwired: 1 in]
                      n59 = Array To Spreadsheet String(array=w189, 3:"%#g" ("format string")) -> (spreadsheet string=w190:string)  [unwired: 1 in]
                      n60 = Format Into String(format string="%d\t%s\n", initial string=w198, error in=w195, w193, w190) -> (resulting string=w197:string, error out=w194:errorcluster)
                    }
                  }
                }
                n61 = Write to Text File(prompt (Choose or enter file path)=w160, text=w166, error in=w165) -> (refnum out=w163:refnum<file>, error out=w164:errorcluster)  [unwired: 1 in, 1 out]
                n62 = Close File(refnum=w163, error in=w164) -> (path=w161:path, error out=w162:errorcluster)
              }
            }
          }
        }
        n63 = in-place-dvr #1() -> (w12:refnum<data-value>, w11:errorcluster)  [unwired: 1 in]
      }
      n64 = Merge Errors(w11, w10) -> (w9:errorcluster)
      n65 = Format Into String(format string=" saved to %s.", initial string=w14, error in=w9, w16) -> (resulting string=w17:string, error out=w18:errorcluster)
    }
    frame Error {
    }
  }
  "error out" <- w4
  "AlliGator IV DVR out" <- w6
  "Message" <- w1
